vi "BRig_dataLC_Reward_Prob_l1.vi"() -> (2 "output_Reward_Prob":i32)   [LabVIEW 2014]
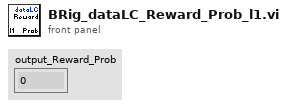
[diagram p1: front panel]
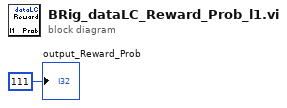
[diagram p0: block diagram]
diagram:
  "output_Reward_Prob" <- 111 ("output_iBlock")
